vi "log analysis_gps.vi"() -> ()   [LabVIEW 2018] (continued)
-15.574401855,0.0,0.757817268,1.584750891,\"631T\",22,13,13,10,04,00,30,33*2671cfe0\n\tsystem status\tnormal 2 28.200000 0 0\trobot status\t31.566635\t41.045143\t9.231100\t-0.643525\t-0.931068\t52.416351\t0.448000\t-0.069000\n\t\n15:07:21.2\tlog_raw\tgps_raw\t#INSPVAXA,USB3,0,44.5,FINESTEERING,2107,281259.200,02000000,471d,15824;INS_ALIGNMENT_COMPLETE,INS_RTKFIXED,37.37050172881,126.72119309205,9.2293,22.3000,0.3645,0.2781,0.0053,-0.664590657,-1.103713757,34.708593103,0.4125,0.2928,0.5558,0.1115,0.0923,0.0801,0.2762,0.2590,5.0316,0f000001,0*10acd44c\n\tsystem status\tnormal 2 28.200000 0 0\trobot status\t31.709898\t41.234302\t9.229300\t-0.664591\t-1.103714\t53.022839\t0.470000\t-0.036000\n\t\n15:07:21.7\tlog_raw\tgps_raw\t#DUALANTENNAHEADINGA,USB3,0,44.5,FINESTEERING,2107,281259.700,02000000,d426,15824;SOL_COMPUTED,NARROW_INT,-1.000000000,37.724102020,-13.091491699,0.0,0.801039636,1.911924362,\"631T\",23,13,13,10,04,00,30,33*9a10e697\n\tsystem status\tnormal 2 28.200000 0 0\trobot status\t31.851856\t41.417794\t9.226400\t-0.835743\t-0.958959\t52.275898\t0.582000\t0.104000\n\t\n15:07:22.2\tlog_raw\tgps_raw\t#DUALANTENNAHEADINGA,USB3,0,46.0,FINESTEERING,2107,281260.200,02000000,d426,15824;SOL_COMPUTED,NARROW_INT,-1.000000000,39.115306854,-14.136718750,0.0,0.803064227,1.840907216,\"631T\",22,13,13,10,04,00,30,33*b50651c8\n\tsystem status\tnormal 2 28.200000 0 0\trobot status\t31.998440\t41.599620\t9.220500\t-0.986235\t-0.919071\t50.884693\t0.455000\t-0.083000\n\t\n15:07:22.7\tlog_raw\tgps_raw\t#INSPVAXA,USB3,0,46.0,FINESTEERING,2107,281260.700,02000000,471d,15824;INS_ALIGNMENT_COMPLETE,INS_RTKFIXED,37.37050659731,126.72119803894,9.2129,22.3000,0.3476,0.2954,-0.0046,-0.736337241,-0.866215786,36.967370061,0.4129,0.2931,0.5580,0.1111,0.0922,0.0796,0.2761,0.2587,5.0324,0f000001,0*f680867e\n\tsystem status\tnormal 2 28.200000 0 0\trobot status\t32.148086\t41.774629\t9.212900\t-0.736337\t-0.866216\t50.520088\t0.373000\t-0.188000\n\t\n15:07:23.2\tlog_raw\tgps_raw\t#DUALANTENNAHEADINGA,USB3,0,47.0,FINESTEERING,2107,281261.200,02000000,d426,15824;SOL_COMPUTED,NARROW_INT,-1.000000000,40.638893127,-14.791442871,0.0,0.948415875,1.839464903,\"631T\",22,13,13,10,04,00,30,33*e03d9ee2\n\tsystem status\tnormal 2 28.200000 0 0\trobot status\t32.299493\t41.952653\t9.205900\t-0.997560\t-1.091665\t49.361107\t0.437000\t-0.086000\n\t\n15:07:23.7\tlog_raw\tgps_raw\t#DUALANTENNAHEADINGA,USB3,0,47.0,FINESTEERING,2107,281261.700,02000000,d426,15824;SOL_COMPUTED,NARROW_INT,-1.000000000,41.109539032,-15.221740723,0.0,0.905525208,1.730005383,\"631T\",23,13,13,10,04,00,30,33*024d4917\n\tsystem status\tnormal 2 28.200000 0 0\trobot status\t32.455230\t42.129270\t9.201000\t-0.840900\t-1.049575\t48.890461\t0.564000\t0.092000\n\t\n15:07:24.2\tlog_raw\tgps_raw\t#INSPVAXA,USB3,0,48.5,FINESTEERING,2107,281262.200,02000000,471d,15824;INS_ALIGNMENT_COMPLETE,INS_RTKFIXED,37.37051135322,126.72120322169,9.1946,22.3000,0.3493,0.3226,-0.0187,-1.003564380,-0.949445467,38.532803613,0.4120,0.2907,0.5583,0.1108,0.0918,0.0785,0.2758,0.2584,5.0341,0f000001,0*bc77f761\n\tsystem status\tnormal 2 28.200000 0 0\trobot status\t32.607165\t42.302460\t9.194600\t-1.003564\t-0.949445\t48.849819\t0.509000\t0.011000\n\t\n15:07:24.7\tlog_raw\tgps_raw\t#DUALANTENNAHEADINGA,USB3,0,48.5,FINESTEERING,2107,281262.700,02000000,d426,15824;SOL_COMPUTED,NARROW_INT,-1.000000000,41.024471283,-13.771057129,0.0,0.941205680,1.970374942,\"631T\",22,13,13,10,04,00,30,33*2b107b4d\n\tsystem status\tnormal 2 28.200000 0 0\trobot status\t32.758480\t42.472024\t9.185100\t-0.965498\t-1.104615\t48.975529\t0.471000\t-0.009000\n\t\n15:07:25.2\tlog_raw\tgps_raw\t#INSPVAXA,USB3,0,45.5,FINESTEERING,2107,281263.200,02000000,471d,15824;INS_ALIGNMENT_COMPLETE,INS_RTKFIXED,37.37051438675,126.72120667905,9.1791,22.3000,0.3385,0.3277,0.0132,-0.749117776,-1.036053021,39.114622535,0.4097,0.2867,0.5508,0.1108,0.0917,0.0777,0.2757,0.2582,5.0350,0f000001,0*900f5f81\n\tsystem status\tnormal 2 28.200000 0 0\trobot status\t32.913413\t42.639134\t9.179100\t-0.749118\t-1.036053\t48.444920\t0.503000\t0.007000\n\t\n15:07:25.7\tlog_raw\tgps_raw\t#INSPVAXA,USB3,0,45.5,FINESTEERING,2107,281263.700,02000000,471d,15824;INS_ALIGNMENT_COMPLETE,INS_RTKFIXED,37.37051592724,126.72120843066,9.1725,22.3000,0.3345,0.3100,-0.0269,-0.953062315,-1.001119813,39.367076268,0.4097,0.2867,0.5508,0.1108,0.0917,0.0777,0.2757,0.2582,5.0350,0f000001,0*3f1ff118\n\tsystem status\tnormal 2 28.200000 0 0\trobot status\t33.068567\t42.810104\t9.172500\t-0.953062\t-1.001120\t48.758610\t0.495000\t0.014000\n\t\n15:07:26.2\tlog_raw\tgps_raw\t#DUALANTENNAHEADINGA,USB3,0,45.5,FINESTEERING,2107,281264.200,02000000,d426,15824;SOL_COMPUTED,NARROW_INT,-1.000000000,41.910186768,-13.638671875,0.0,0.987370729,2.013862848,\"631T\",24,13,13,10,04,00,30,33*886cbc18\n\tsystem status\tnormal 2 28.200000 0 0\trobot status\t33.222421\t42.973971\t9.165800\t-0.908836\t-0.953888\t48.089813\t0.490000\t0.012000\n\t\n15:07:26.7\tlog_raw\tgps_raw\t#DUALANTENNAHEADINGA,USB3,0,45.5,FINESTEERING,2107,281264.700,02000000,d426,15824;SOL_COMPUTED,NARROW_INT,-1.000000000,42.165882111,-13.191467285,0.0,1.231637120,2.283805132,\"631T\",23,11,11,8,04,00,30,03*d347cf5b\n\tsystem status\tnormal 2 28.200000 0 0\trobot status\t33.385986\t43.147920\t9.157400\t-0.806230\t-0.977712\t47.834118\t0.498000\t0.015000\n\t\n15:07:27.2\tlog_raw\tgps_raw\t#DUALANTENNAHEADINGA,USB3,0,48.5,FINESTEERING,2107,281265.200,02000000,d426,15824;SOL_COMPUTED,NARROW_INT,-1.000000000,41.782566071,-14.026184082,0.0,0.949394464,1.456767678,\"631T\",24,12,12,8,04,00,30,03*b5e68f03\n\tsystem status\tnormal 2 28.300000 0 0\trobot status\t33.551266\t43.323593\t9.149800\t-0.943344\t-1.087324\t48.217434\t0.504000\t0.015000\n\t\n15:07:27.7\tlog_raw\tgps_raw\t#DUALANTENNAHEADINGA,USB3,0,48.5,FINESTEERING,2107,281265.700,02000000,d426,15824;SOL_COMPUTED,NARROW_INT,-1.000000000,42.654987335,-13.940582275,0.0,0.905997872,1.456194401,\"631T\",25,12,12,8,04,00,30,03*ebbb69a1\n\tsystem status\tnormal 2 28.200000 0 0\trobot status\t33.713510\t43.493528\t9.144600\t-0.914763\t-1.022784\t47.345013\t0.602000\t-0.140000\n\t\n15:07:28.2\tlog_raw\tgps_raw\t#DUALANTENNAHEADINGA,USB3,0,44.0,FINESTEERING,2107,281266.200,02000000,d426,15824;SOL_COMPUTED,NARROW_INT,-1.000000000,41.473289490,-13.976562500,0.0,0.876108646,1.437642574,\"631T\",26,12,12,8,04,00,30,03*9c4cfbf2\n\tsystem status\tnormal 2 28.100000 0 0\trobot status\t33.872849\t43.664287\t9.139200\t-0.953588\t-0.975012\t48.526711\t0.573000\t-0.084000\n\t\n15:07:28.7\tlog_raw\tgps_raw\t#INSPVAXA,USB3,0,44.0,FINESTEERING,2107,281266.700,02000000,471d,15824;INS_ALIGNMENT_COMPLETE,INS_RTKFIXED,37.37052514721,126.72121924696,9.1351,22.3000,0.3260,0.3161,-0.0126,-0.947375074,-0.706024295,38.522505124,0.4363,0.2885,0.5509,0.1172,0.0950,0.0803,0.2752,0.2577,5.0353,0f000001,0*ab36857c\n\tsystem status\tnormal 2 28.000000 0 0\trobot status\t34.026658\t43.833375\t9.135100\t-0.947375\t-0.706024\t48.338646\t0.361000\t0.243000\n\t\n15:07:29.2\tlog_raw\tgps_raw\t#DUALANTENNAHEADINGA,USB3,0,48.0,FINESTEERING,2107,281267.200,02000000,d426,15824;SOL_COMPUTED,NARROW_INT,-1.000000000,40.023796082,-13.769653320,0.0,1.105050921,2.107353687,\"631T\",22,12,12,8,04,00,30,03*89f55c6d\n\tsystem status\tnormal 2 28.000000 0 0\trobot status\t34.180182\t44.006389\t9.131600\t-0.895036\t-0.801690\t49.976204\t0.562000\t-0.071000\n\t\n15:07:29.7\tlog_raw\tgps_raw\t#DUALANTENNAHEADINGA,USB3,0,48.0,FINESTEERING,2107,281267.700,02000000,d426,15824;SOL_COMPUTED,NARROW_INT,-1.000000000,38.975990295,-14.866943359,0.0,1.019285679,1.869416475,\"631T\",22,12,12,8,04,00,30,03*a0488b34\n\tsystem status\tnormal 2 28.000000 0 0\trobot status\t34.334172\t44.181531\t9.127500\t-0.727606\t-0.705041\t51.024010\t0.354000\t0.251000\n\t\n15:07:30.2\tlog_raw\tgps_raw\t#DUALANTENNAHEADINGA,USB3,0,48.0,FINESTEERING,2107,281268.200,02000000,d426,15824;SOL_COMPUTED,NARROW_INT,-1.000000000,37.457145691,-14.142669678,0.0,0.916966915,1.645377994,\"631T\",25,12,12,8,04,00,30,03*51ae3b94\n\tsystem status\tnormal 2 28.000000 0 0\trobot status\t34.484633\t44.363511\t9.124000\t-0.782242\t-1.013218\t52.542854\t0.617000\t-0.117000\n\t\n15:07:30.7\tlog_raw\tgps_raw\t#DUALANTENNAHEADINGA,USB3,0,48.0,FINESTEERING,2107,281268.700,02000000,d426,15824;SOL_COMPUTED,NARROW_INT,-1.000000000,36.570995331,-12.889495850,0.0,0.874405205,1.610776067,\"631T\",27,12,12,8,04,00,30,03*59172eb5\n\tsystem status\tnormal 2 28.000000 0 0\trobot status\t34.629130\t44.546597\t9.120400\t-0.707911\t-0.956168\t53.429005\t0.665000\t-0.257000\n\t\n15:07:31.2\tlog_raw\tgps_raw\t#DUALANTENNAHEADINGA,USB3,0,43.5,FINESTEERING,2107,281269.200,02000000,d426,15824;SOL_COMPUTED,NARROW_INT,-1.000000000,35.973979950,-14.332061768,0.0,0.830094159,1.497864485,\"631T\",27,12,12,8,04,00,30,03*090ddc0d\n\tsystem status\tnormal 2 28.100000 0 0\trobot status\t34.770052\t44.733261\t9.118400\t-0.795683\t-0.850425\t54.026020\t0.605000\t-0.143000\n\t\n15:07:31.7\tlog_raw\tgps_raw\t#DUALANTENNAHEADINGA,USB3,0,43.5,FINESTEERING,2107,281269.700,02000000,d426,15824;SOL_COMPUTED,NARROW_INT,-1.000000000,35.818984985,-16.138092041,0.0,0.812042832,1.471114397,\"631T\",26,12,12,8,04,00,30,03*f4bb3c31\n\tsystem status\tnormal 2 28.100000 0 0\trobot status\t34.908478\t44.923072\t9.116600\t-0.660770\t-0.782310\t54.181015\t0.442000\t0.104000\n\t\n15:07:32.2\tlog_raw\tgps_raw\t#DUALANTENNAHEADINGA,USB3,0,46.5,FINESTEERING,2107,281270.200,02000000,d426,15824;SOL_COMPUTED,NARROW_INT,-1.000000000,35.621791840,-13.436737061,0.0,0.778346181,1.418952346,\"631T\",25,12,12,8,04,00,30,03*c6e6dbb2\n\tsystem status\tnormal 2 28.100000 0 0\trobot status\t35.047785\t45.119572\t9.114200\t-0.835759\t-0.956556\t54.378208\t0.421000\t0.108000\n\t\n15:07:32.7\tlog_raw\tgps_raw\t#DUALANTENNAHEADINGA,USB3,0,46.5,FINESTEERING,2107,281270.700,02000000,d426,15824;SOL_COMPUTED,NARROW_INT,-1.000000000,35.070240021,-13.728149414,0.0,0.744003534,1.356679201,\"631T\",25,12,12,8,04,00,30,03*cf10d1c9\n\tsystem status\tnormal 2 28.200000 0 0\trobot status\t35.184021\t45.314772\t9.112900\t-0.827370\t-0.902708\t54.929760\t0.608000\t-0.143000\n\t\n15:07:33.2\tlog_raw\tgps_raw\t#DUALANTENNAHEADINGA,USB3,0,45.5,FINESTEERING,2107,281271.200,02000000,d426,15824;SOL_COMPUTED,NARROW_INT,-1.000000000,35.494377136,-13.422943115,0.0,0.983616889,2.186612129,\"631T\",23,12,12,8,04,00,30,03*afbd86f5\n\tsystem status\tnormal 2 28.200000 0 0\trobot status\t35.321899\t45.512581\t9.111000\t-0.616810\t-0.962309\t54.505623\t0.386000\t0.164000\n\t\n15:07:33.7\tlog_raw\tgps_raw\t#DUALANTENNAHEADINGA,USB3,0,45.5,FINESTEERING,2107,281271.700,02000000,d426,15824;SOL_COMPUTED,NARROW_INT,-1.000000000,35.115871429,-12.229492188,0.0,0.917624831,2.129554033,\"631T\",22,11,11,8,04,00,30,03*47d1ca67\n\tsystem status\tnormal 2 28.200000 0 0\trobot status\t35.456033\t45.711150\t9.110300\t-0.770202\t-0.898350\t54.884129\t0.467000\t0.040000\n\t\n15:07:34.2\tlog_raw\tgps_raw\t#DUALANTENNAHEADINGA,USB3,0,45.0,FINESTEERING,2107,281272.200,02000000,d426,15824;SOL_COMPUTED,NARROW_INT,-1.000000000,35.165107727,-13.680572510,0.0,0.853601813,1.895400286,\"631T\",23,11,11,8,04,00,30,03*664b8012\n\tsystem status\tnormal 2 28.200000 0 0\trobot status\t35.595153\t45.913396\t9.108200\t-0.692435\t-1.007162\t54.834892\t0.467000\t0.023000\n\t\n15:07:34.7\tlog_raw\tgps_raw\t#DUALANTENNAHEADINGA,USB3,0,45.0,FINESTEERING,2107,281272.700,02000000,d426,15824;SOL_COMPUTED,NARROW_INT,-1.000000000,35.308296204,-13.433410645,0.0,0.833106577,1.789978504,\"631T\",23,11,11,8,04,00,30,03*efeaf6da\n\tsystem status\tnormal 2 28.200000 0 0\trobot status\t35.734434\t46.115790\t9.102900\t-0.678981\t-1.146702\t54.691704\t0.482000\t0.009000\n\t\n15:07:35.2\tlog_raw\tgps_raw\t#DUALANTENNAHEADINGA,USB3,0,46.0,FINESTEERING,2107,281273.200,02000000,d426,15824;SOL_COMPUTED,NARROW_INT,-1.000000000,36.192741394,-16.037811279,0.0,0.810550869,1.694264531,\"631T\",22,11,11,8,04,00,30,03*4456d48d\n\tsystem status\tnormal 2 28.200000 0 0\trobot status\t35.871255\t46.311320\t9.099300\t-0.536086\t-1.483888\t53.807259\t0.505000\t-0.028000\n\t\n15:07:35.7\tlog_raw\tgps_raw\t\tsystem status\tnormal 2 28.200000 0 0\trobot status\t36.007822\t46.507939\t9.097500\t-0.602065\t-1.516155\t53.983997\t0.489000\t-0.023000\n\t\n15:07:36.2\tlog_raw\tgps_raw\t#DUALANTENNAHEADINGA,USB3,0,48.0,FINESTEERING,2107,281274.200,02000000,d426,15824;SOL_COMPUTED,NARROW_INT,-1.000000000,35.622310638,-14.246795654,0.0,1.186534643,2.124257803,\"631T\",23,13,13,10,04,00,30,33*4699dedc\n\tsystem status\tnormal 2 28.200000 0 0\trobot status\t36.147250\t46.710270\t9.090800\t-0.727838\t-1.235927\t54.377689\t0.492000\t-0.015000\n\t\n15:07:36.7\tlog_raw\tgps_raw\t\tsystem status\tnormal 2 28.300000 0 0\trobot status\t36.284167\t46.907030\t9.084300\t-0.725999\t-1.253532\t54.463184\t0.493000\t-0.018000\n\t\n15:07:37.2\tlog_raw\tgps_raw\t#DUALANTENNAHEADINGA,USB3,0,45.0,FINESTEERING,2107,281275.200,02000000,d426,15824;SOL_COMPUTED,NARROW_INT,-1.000000000,35.922065735,-12.943084717,0.0,1.068319321,2.159161329,\"631T\",24,13,13,10,04,00,30,23*90535b08\n\tsystem status\tnormal 2 28.300000 0 0\trobot status\t36.415424\t47.091111\t9.080700\t-0.590725\t-1.108653\t54.077934\t0.494000\t-0.024000\n\t\n15:07:37.7\tlog_raw\tgps_raw\t#DUALANTENNAHEADINGA,USB3,0,45.0,FINESTEERING,2107,281275.700,02000000,d426,15824;SOL_COMPUTED,NARROW_INT,-1.000000000,35.806697845,-14.127471924,0.0,1.191707134,2.929863453,\"631T\",23,13,13,10,04,00,30,33*14f638f6\n\tsystem status\tnormal 2 28.200000 0 0\trobot status\t36.555534\t47.288330\t9.077900\t-0.847597\t-1.031601\t54.193302\t0.498000\t-0.035000\n\t\n15:07:38.2\tlog_raw\tgps_raw\t\tsystem status\tnormal 2 28.200000 0 0\trobot status\t36.697376\t47.486132\t9.075700\t-0.966277\t-0.867460\t53.488716\t0.476000\t-0.014000\n\t\n15:07:38.7\tlog_raw\tgps_raw\t\tsystem status\tnormal 2 28.200000 0 0\trobot status\t36.838734\t47.678234\t9.075000\t-0.743731\t-0.878510\t52.994225\t0.507000\t-0.012000\n\t\n15:07:39.2\tlog_raw\tgps_raw\t#DUALANTENNAHEADINGA,USB3,0,47.5,FINESTEERING,2107,281277.200,02000000,d426,15824;SOL_COMPUTED,NARROW_INT,-1.000000000,36.727424622,-13.082946777,0.0,0.949807763,2.157425642,\"631T\",23,11,11,8,04,00,30,03*dbda4352\n\tsystem status\tnormal 2 28.200000 0 0\trobot status\t36.981502\t47.872071\t9.074100\t-0.771341\t-0.814677\t53.272575\t0.497000\t-0.019000\n\t\n15:07:39.7\tlog_raw\tgps_raw\t\tsystem status\tnormal 2 28.200000 0 0\trobot status\t37.126902\t48.063305\t9.075700\t-0.664587\t-1.042074\t53.167221\t0.578000\t0.099000\n\t\n15:07:40.2\tlog_raw\tgps_raw\t#DUALANTENNAHEADINGA,USB3,0,47.0,FINESTEERING,2107,281278.200,02000000,d426,15824;SOL_COMPUTED,NARROW_INT,-1.000000000,38.801025391,-13.665405273,0.0,1.011600971,2.213801622,\"631T\",23,11,11,8,04,00,30,03*a2b4300d\n\tsystem status\tnormal 2 28.200000 0 0\trobot status\t37.270479\t48.250911\t9.075300\t-0.703013\t-0.987348\t51.198975\t0.484000\t-0.048000\n\t\n15:07:40.7\tlog_raw\tgps_raw\t\tsystem status\tnormal 2 28.200000 0 0\trobot status\t37.419608\t48.442360\t9.072100\t-0.758993\t-1.063474\t50.790871\t0.434000\t-0.124000\n\t\n15:07:41.2\tlog_raw\tgps_raw\t#DUALANTENNAHEADINGA,USB3,0,44.5,FINESTEERING,2107,281279.200,02000000,d426,15824;SOL_COMPUTED,NARROW_INT,-1.000000000,39.271907806,-13.744201660,0.0,0.885574758,1.866288543,\"631T\",24,11,11,8,04,00,30,03*14651a74\n\tsystem status\tnormal 2 28.200000 0 0\trobot status\t37.564073\t48.625273\t9.068400\t-0.756006\t-0.992828\t50.728092\t0.460000\t-0.070000\n\t\n15:07:41.7\tlog_raw\tgps_raw\t\tsystem status\tnormal 2 28.200000 0 0\trobot status\t37.713760\t48.813692\t9.062800\t-0.823894\t-1.057064\t50.037521\t0.395000\t-0.114000\n\t\n15:07:42.2\tlog_raw\tgps_raw\t\tsystem status\tnormal 2 28.200000 0 0\trobot status\t37.862921\t48.995193\t9.058900\t-0.752662\t-0.902912\t50.282597\t0.502000\t0.016000\n\t\n15:07:42.7\tlog_raw\tgps_raw\t#DUALANTENNAHEADINGA,USB3,0,48.0,FINESTEERING,2107,281280.700,02000000,d426,15824;SOL_COMPUTED,NARROW_INT,-1.000000000,40.700374603,-12.203552246,0.0,0.796584129,1.643284798,\"631T\",24,11,11,8,04,00,30,03*0355bfc3\n\tsystem status\tnormal 2 28.200000 0 0\trobot status\t38.015447\t49.176889\t9.058400\t-0.805111\t-0.901408\t49.299625\t0.476000\t-0.022000\n\t\n15:07:43.2\tlog_raw\tgps_raw\t\tsystem status\tnormal 2 28.200000 0 0\trobot status\t38.168522\t49.355987\t9.054400\t-0.980266\t-0.609275\t49.185120\t0.511000\t0.011000\n\t\n15:07:43.7\tlog_raw\tgps_raw\t#DUALANTENNAHEADINGA,USB3,0,43.5,FINESTEERING,2107,281281.700,02000000,d426,15824;SOL_COMPUTED,NARROW_INT,-1.000000000,41.025180817,-13.610565186,0.0,1.006764770,1.762146711,\"631T\",23,11,11,8,04,00,30,03*95eb9222\n\tsystem status\tnormal 2 28.200000 0 0\trobot status\t38.323525\t49.525802\t9.048900\t-0.595366\t-0.860197\t48.974819\t0.485000\t0.004000\n\t\n15:07:44.2\tlog_raw\tgps_raw\t\tsystem status\tnormal 2 28.200000 0 0\trobot status\t38.479198\t49.700891\t9.045700\t-0.786808\t-0.739360\t47.852482\t0.490000\t0.014000\n\t\n15:07:44.7\tlog_raw\tgps_raw\t#DUALANTENNAHEADINGA,USB3,0,48.5,FINESTEERING,2107,281282.700,02000000,d426,15824;SOL_COMPUTED,NARROW_INT,-1.000000000,42.471115112,-14.988128662,0.0,1.268621087,2.738634586,\"631T\",23,13,13,9,04,00,20,23*7676e672\n\tsystem status\tnormal 2 28.200000 0 0\trobot status\t38.628012\t49.869703\t9.041100\t-1.082338\t-0.662611\t47.528885\t0.491000\t0.015000\n\t\n15:07:45.2\tlog_raw\tgps_raw\t#INSPVAXA,USB3,0,48.0,FINESTEERING,2107,281283.250,02000000,471d,15824;INS_ALIGNMENT_COMPLETE,INS_RTKFIXED,37.37058125614,126.72127316558,9.0365,22.3000,0.3478,0.3335,-0.0027,-0.704403404,-0.836236554,39.118701803,0.4319,0.3133,0.6216,0.1204,0.1024,0.0974,0.2734,0.2534,5.0561,0f000001,0*0df7e601\n\tsystem status\tnormal 2 28.200000 0 0\trobot status\t38.802681\t50.060581\t9.036500\t-0.704403\t-0.836237\t48.533897\t0.502000\t0.030000\n\t\n15:07:45.7\tlog_raw\tgps_raw\t#DUALANTENNAHEADINGA,USB3,0,48.0,FINESTEERING,2107,281283.700,02000000,d426,15824;SOL_COMPUTED,NARROW_INT,-1.000000000,41.292312622,-13.761383057,0.0,1.487377644,3.398363352,\"631T\",25,10,10,8,04,00,30,03*49b52b61\n\tsystem status\tnormal 2 28.200000 0 0\trobot status\t38.946357\t50.221947\t9.035600\t-0.938084\t-0.748688\t48.707687\t0.500000\t0.017000\n\t\n15:07:46.2\tlog_raw\tgps_raw\t#INSPVAXA,USB3,0,44.5,FINESTEERING,2107,281284.250,02000000,471d,15824;INS_ALIGNMENT_COMPLETE,INS_RTKFIXED,37.37058446322,126.72127677415,9.0328,22.3000,0.3259,0.3273,-0.0037,-0.937814691,-0.658439283,39.092377906,0.4304,0.3133,0.6248,0.1182,0.0996,0.0951,0.2734,0.2534,5.0568,0f000001,0*6df0d0a0\n\tsystem status\tnormal 2 28.200000 0 0\trobot status\t39.122322\t50.416516\t9.032800\t-0.937815\t-0.658439\t49.048512\t0.434000\t0.108000\n\t\n15:07:46.7\tlog_raw\tgps_raw\t\tsystem status\tnormal 2 28.100000 0 0\trobot status\t39.265720\t50.576645\t9.028100\t-0.931821\t-0.651062\t48.507782\t0.516000\t-0.019000\n\t\n15:07:47.2\tlog_raw\tgps_raw\t#DUALANTENNAHEADINGA,USB3,0,45.0,FINESTEERING,2107,281285.200,02000000,d426,15824;SOL_COMPUTED,NARROW_INT,-1.000000000,40.100524902,-11.947021484,0.0,1.414593220,3.733982325,\"631T\",25,10,10,8,04,00,30,03*9b9ac519\n\tsystem status\tnormal 2 28.100000 0 0\trobot status\t39.418438\t50.753731\t9.026400\t-1.045904\t-0.622362\t49.899475\t0.367000\t0.232000\n\t\n15:07:47.7\tlog_raw\tgps_raw\t#INSPVAXA,USB3,0,45.0,FINESTEERING,2107,281285.750,02000000,471d,15824;INS_ALIGNMENT_COMPLETE,INS_RTKFIXED,37.37058925318,126.72128198037,9.0239,22.3000,0.3334,0.2935,0.0143,-0.808488626,-0.666784324,37.099598741,0.4334,0.3188,0.6428,0.1170,0.0987,0.0941,0.2735,0.2534,5.0574,0f000001,0*332dca9d\n\tsystem status\tnormal 2 28.100000 0 0\trobot status\t39.583480\t50.948126\t9.023900\t-0.808489\t-0.666784\t50.980686\t0.340000\t0.231000\n\t\n15:07:48.2\tlog_raw\tgps_raw\t\tsystem status\tnormal 2 28.000000 0 0\trobot status\t39.716456\t51.111886\t9.021500\t-0.669660\t-0.741115\t51.504147\t0.461000\t0.100000\n\t\n15:07:48.7\tlog_raw\tgps_raw\t#DUALANTENNAHEADINGA,USB3,0,47.0,FINESTEERING,2107,281286.700,02000000,d426,15824;SOL_COMPUTED,NARROW_INT,-1.000000000,38.718589783,-13.239685059,0.0,1.092944860,2.696835995,\"631T\",24,10,10,8,04,00,30,03*03484901\n\tsystem status\tnormal 2 28.000000 0 0\trobot status\t39.859819\t51.303062\t9.018200\t-0.911625\t-1.044323\t51.281410\t0.609000\t-0.142000\n\t\n15:07:49.2\tlog_raw\tgps_raw\t\tsystem status\tnormal 2 28.000000 0 0\trobot status\t39.998635\t51.492159\t9.013800\t-0.809440\t-1.050845\t52.888622\t0.391000\t0.170000\n\t\n15:07:49.7\tlog_raw\tgps_raw\t#DUALANTENNAHEADINGA,USB3,0,47.0,FINESTEERING,2107,281287.700,02000000,d426,15824;SOL_COMPUTED,NARROW_INT,-1.000000000,36.104297638,-13.498443604,0.0,0.922848761,2.195329189,\"631T\",26,10,10,8,04,00,30,03*04480a52\n\tsystem status\tnormal 2 28.100000 0 0\trobot status\t40.135370\t51.683837\t9.009000\t-0.800921\t-0.896046\t53.895702\t0.367000\t0.224000\n\t\n15:07:50.2\tlog_raw\tgps_raw\t#INSPVAXA,USB3,0,47.5,FINESTEERING,2107,281288.250,02000000,471d,15824;INS_ALIGNMENT_COMPLETE,INS_RTKFIXED,37.37059781001,126.72128984433,9.0038,22.3000,0.3744,0.2594,-0.0022,-0.807848341,-0.697649833,32.607000206,0.4351,0.3197,0.6721,0.1156,0.0982,0.0924,0.2733,0.2531,5.0607,0f000001,0*7ad3d381\n\tsystem status\tnormal 2 28.100000 0 0\trobot status\t40.280057\t51.897799\t9.003800\t-0.807848\t-0.697650\t53.988251\t0.428000\t0.116000\n\t\n15:07:50.7\tlog_raw\tgps_raw\t#DUALANTENNAHEADINGA,USB3,0,47.5,FINESTEERING,2107,281288.700,02000000,d426,15824;SOL_COMPUTED,NARROW_INT,-1.000000000,34.380798340,-12.289306641,0.0,0.881599903,2.027381897,\"631T\",24,10,10,8,04,00,30,03*fd23ace1\n\tsystem status\tnormal 2 28.100000 0 0\trobot status\t40.398568\t52.080059\t8.999400\t-0.727871\t-0.931697\t55.619202\t0.598000\t-0.139000\n\t\n15:07:51.2\tlog_raw\tgps_raw\t#INSPVAXA,USB3,0,43.0,FINESTEERING,2107,281289.250,02000000,471d,15824;INS_ALIGNMENT_COMPLETE,INS_RTKFIXED,37.37060144846,126.72129278207,8.9959,22.3000,0.3637,0.2540,-0.0055,-0.784801364,-1.198337190,31.676492197,0.4344,0.3185,0.6737,0.1148,0.0977,0.0905,0.2732,0.2529,5.0623,0f000001,0*0e64d244\n\tsystem status\tnormal 2 28.100000 0 0\trobot status\t40.540277\t52.301609\t8.995900\t-0.784801\t-1.198337\t55.390762\t0.568000\t-0.112000\n\t\n15:07:51.7\tlog_raw\tgps_raw\t\tsystem status\tnormal 2 28.200000 0 0\trobot status\t40.656983\t52.485859\t8.990900\t-0.841622\t-1.206879\t55.521332\t0.426000\t0.109000\n\t\n15:07:52.2\tlog_raw\tgps_raw\t#DUALANTENNAHEADINGA,USB3,0,47.0,FINESTEERING,2107,281290.200,02000000,d426,15824;SOL_COMPUTED,NARROW_INT,-1.000000000,34.493209839,-14.783813477,0.0,0.972535849,1.987741113,\"631T\",22,10,10,8,04,00,30,03*2d07aef6\n\tsystem status\tnormal 2 28.200000 0 0\trobot status\t40.786858\t52.689235\t8.985800\t-0.708265\t-1.382941\t55.506790\t0.550000\t-0.106000\n\t\n15:07:52.7\tlog_raw\tgps_raw\t\tsystem status\tnormal 2 28.200000 0 0\trobot status\t40.919320\t52.896058\t8.981700\t-0.619521\t-1.535397\t55.462795\t0.462000\t0.033000\n\t\n15:07:53.2\tlog_raw\tgps_raw\t#INSPVAXA,USB3,0,47.0,FINESTEERING,2107,281291.250,02000000,471d,15824;INS_ALIGNMENT_COMPLETE,INS_RTKFIXED,37.37060884718,126.72129871265,8.9767,22.3000,0.3938,0.2598,0.0143,-0.672164734,-1.279451684,31.580297519,0.4248,0.3046,0.6381,0.1143,0.0969,0.0864,0.2729,0.2527,5.0655,0f000001,0*eac27b45\n\tsystem status\tnormal 2 28.200000 0 0\trobot status\t41.065598\t53.122751\t8.976700\t-0.672165\t-1.279452\t55.013996\t0.503000\t-0.018000\n\t\n15:07:53.7\tlog_raw\tgps_raw\t\tsystem status\tnormal 2 28.200000 0 0\trobot status\t41.180313\t53.298203\t8.973400\t-0.877294\t-1.135816\t54.990143\t0.474000\t0.003000\n\t\n15:07:54.2\tlog_raw\tgps_raw\t#INSPVAXA,USB3,0,48.0,FINESTEERING,2107,281292.250,02000000,471d,15824;INS_ALIGNMENT_COMPLETE,INS_RTKFIXED,37.37061243778,126.72130169584,8.9693,22.3000,0.3929,0.2526,0.0002,-0.566566315,-1.022014825,31.866570439,0.4222,0.3014,0.6236,0.1151,0.0976,0.0859,0.2728,0.2526,5.0668,0f000001,0*f1faa83c\n\tsystem status\tnormal 2 28.200000 0 0\trobot status\t41.329844\t53.521251\t8.969300\t-0.566566\t-1.022015\t54.607853\t0.494000\t-0.018000\n\t\n15:07:54.7\tlog_raw\tgps_raw\t\tsystem status\tnormal 2 28.200000 0 0\trobot status\t41.448026\t53.700928\t8.965600\t-0.554965\t-1.221563\t55.514385\t0.495000\t-0.016000\n\t\n15:07:55.2\tlog_raw\tgps_raw\t#INSPVAXA,USB3,0,46.5,FINESTEERING,2107,281293.250,02008000,471d,15824;INS_ALIGNMENT_COMPLETE,INS_RTKFIXED,37.37061609007,126.72130472150,8.9616,22.3000,0.3940,0.2710,0.0085,-0.635134028,-1.458627956,32.227180658,0.4201,0.2993,0.6101,0.1147,0.0971,0.0842,0.2727,0.2523,5.0683,0f000001,0*f561f230\n\tsystem status\tnormal 2 28.200000 0 0\trobot status\t41.597852\t53.926597\t8.961600\t-0.635134\t-1.458628\t55.285629\t0.495000\t-0.018000\n\t\n15:07:55.7\tlog_raw\tgps_raw\t\tsystem status\tnormal 2 28.200000 0 0\trobot status\t41.717377\t54.101745\t8.958300\t-0.727505\t-1.117508\t55.508831\t0.490000\t-0.016000\n\t\n15:07:56.2\tlog_raw\tgps_raw\t#INSPVAXA,USB3,0,44.0,FINESTEERING,2107,281294.250,02008000,471d,15824;INS_ALIGNMENT_COMPLETE,INS_RTKFIXED,37.37061971209,126.72130780942,8.9541,22.3000,0.4211,0.2805,-0.0013,-0.831057528,-0.973116306,32.803325503,0.4188,0.2977,0.5988,0.1153,0.0975,0.0844,0.2725,0.2520,5.0696,0f000001,0*1928a823\n\tsystem status\tnormal 2 28.200000 0 0\trobot status\t41.871375\t54.328584\t8.954100\t-0.831058\t-0.973116\t54.554722\t0.492000\t-0.026000\n\t\n15:07:56.7\tlog_raw\tgps_raw\t#INSPVAXA,USB3,0,44.0,FINESTEERING,2107,281294.750,02008000,471d,15824;INS_ALIGNMENT_COMPLETE,INS_RTKFIXED,37.37062151019,126.72130936764,8.9520,22.3000,0.3975,0.2634,0.0090,-0.724790685,-1.060395947,33.026627760,0.4188,0.2977,0.5988,0.1153,0.0975,0.0844,0.2725,0.2520,5.0696,0f000001,0*daa7d020\n\tsystem status\tnormal 2 28.200000 0 0\trobot status\t42.009400\t54.528145\t8.952000\t-0.724791\t-1.060396\t54.415871\t0.495000\t-0.025000\n\t\n15:07:57.2\tlog_raw\tgps_raw\t#INSPVAXA,USB3,0,48.0,FINESTEERING,2107,281295.250,02008000,471d,15824;INS_ALIGNMENT_COMPLETE,INS_RTKFIXED,37.37062331676,126.72131094056,8.9508,22.3000,0.4136,0.2984,0.0031,-0.941558155,-1.233075222,33.345568477,0.4178,0.2964,0.5888,0.1164,0.0983,0.0857,0.2723,0.2516,5.0710,0f000001,0*4b91ac30\n\tsystem status\tnormal 2 28.200000 0 0\trobot status\t42.148726\t54.728646\t8.950800\t-0.941558\t-1.233075\t54.361309\t0.492000\t-0.016000\n\t\n15:07:57.7\tlog_raw\tgps_raw\t#INSPVAXA,USB3,0,48.0,FINESTEERING,2107,281295.750,02008000,471d,15824;INS_ALIGNMENT_COMPLETE,INS_RTKFIXED,37.37062507494,126.72131254716,8.9509,22.3000,0.4055,0.2849,-0.0018,-0.776132833,-1.125745955,33.718162525,0.4178,0.2964,0.5888,0.1164,0.0983,0.0857,0.2723,0.2516,5.0710,0f000001,0*fb568b3d\n\tsystem status\tnormal 2 28.200000 0 0\trobot status\t42.291036\t54.923776\t8.950900\t-0.776133\t-1.125746\t53.586090\t0.505000\t-0.016000\n\t\n15:07:58.2\tlog_raw\tgps_raw\t\tsystem status\tnormal 2 28.200000 0 0\trobot status\t42.419876\t55.099393\t8.950200\t-0.725828\t-1.060978\t53.230602\t0.498000\t-0.023000\n\t\n15:07:58.7\tlog_raw\tgps_raw\t#INSPVAXA,USB3,0,46.0,FINESTEERING,2107,281296.750,02008000,471d,15824;INS_ALIGNMENT_COMPLETE,INS_RTKFIXED,37.37062859977,126.72131581022,8.9479,22.3000,0.4084,0.2870,-0.0048,-0.626858004,-1.220047276,34.496993035,0.4174,0.2953,0.5808,0.1166,0.0980,0.0866,0.2720,0.2512,5.0719,0f000001,0*b70d9a1a\n\tsystem status\tnormal 2 28.200000 0 0\trobot status\t42.580073\t55.314976\t8.947900\t-0.626858\t-1.220047\t52.350243\t0.492000\t-0.024000\n\t\n15:07:59.2\tlog_raw\tgps_raw\t\tsystem status\tnormal 2 28.200000 0 0\trobot status\t42.709665\t55.485973\t8.946000\t-0.724943\t-0.913191\t51.877937\t0.504000\t-0.019000\n\t\n15:07:59.7\tlog_raw\tgps_raw\t#INSPVAXA,USB3,0,46.5,FINESTEERING,2107,281297.750,02000000,471d,15824;INS_ALIGNMENT_COMPLETE,INS_RTKFIXED,37.37063201269,126.72131910032,8.9415,22.3000,0.3858,0.2920,-0.0049,-0.857107455,-1.040274472,35.314316198,0.4170,0.2951,0.5749,0.1163,0.0975,0.0871,0.2718,0.2508,5.0734,0f000001,0*148bd1ed\n\tsystem status\tnormal 2 28.300000 0 0\trobot status\t42.871505\t55.693757\t8.941500\t-0.857107\t-1.040274\t51.127346\t0.541000\t0.060000\n\t\n15:08:00.2\tlog_raw\tgps_raw\t#INSPVAXA,USB3,0,47.5,FINESTEERING,2107,281298.250,02000000,471d,15824;INS_ALIGNMENT_COMPLETE,INS_RTKFIXED,37.37063371305,126.72132080320,8.9374,22.3000,0.3749,0.3041,0.0076,-0.820490736,-1.287497218,35.568330559,0.4168,0.2950,0.5704,0.1159,0.0968,0.0877,0.2716,0.2505,5.0751,0f000001,0*0458b711\n\tsystem status\tnormal 2 28.200000 0 0\trobot status\t43.022343\t55.882470\t8.937400\t-0.820491\t-1.287497\t52.237698\t0.484000\t-0.013000\n\t\n15:08:00.7\tlog_raw\tgps_raw\t\tsystem status\tnormal 2 28.200000 0 0\trobot status\t43.152336\t56.043862\t8.935300\t-0.982494\t-1.398492\t50.827724\t0.480000\t-0.007000\n\t\n15:08:01.2\tlog_raw\tgps_raw\t#INSPVAXA,USB3,0,48.0,FINESTEERING,2107,281299.250,02000000,471d,15824;INS_ALIGNMENT_COMPLETE,INS_RTKFIXED,37.37063695179,126.72132414290,8.9320,22.3000,0.3767,0.2972,0.0004,-0.739787726,-1.092581403,36.370475984,0.4162,0.2936,0.5661,0.1155,0.0962,0.0881,0.2714,0.2503,5.0767,0f000001,0*980b2911\n\tsystem status\tnormal 2 28.200000 0 0\trobot status\t43.318168\t56.241918\t8.932000\t-0.739788\t-1.092581\t51.898197\t0.494000\t-0.011000\n\t\n15:08:01.7\tlog_raw\tgps_raw\t#INSPVAXA,USB3,0,48.0,FINESTEERING,2107,281299.750,02000000,471d,15824;INS_ALIGNMENT_COMPLETE,INS_RTKFIXED,37.37063857725,126.72132585702,8.9270,22.3000,0.3719,0.3148,0.0043,-0.737895433,-1.223503382,36.673164573,0.4162,0.2936,0.5661,0.1155,0.0962,0.0881,0.2714,0.2503,5.0767,0f000001,0*b3e17f59\n\tsystem status\tnormal 2 28.200000 0 0\trobot status\t43.470002\t56.422319\t8.927000\t-0.737895\t-1.223503\t51.044170\t0.499000\t0.000000\n\t\n15:08:02.2\tlog_raw\tgps_raw\t\tsystem status\tnormal 2 28.200000 0 0\trobot status\t43.603521\t56.579476\t8.926700\t-0.766315\t-1.182755\t50.454479\t0.491000\t0.011000\n\t\n15:08:02.7\tlog_raw\tgps_raw\t#INSPVAXA,USB3,0,49.0,FINESTEERING,2107,281300.750,02000000,471d,15824;INS_ALIGNMENT_COMPLETE,INS_RTKFIXED,37.37064174008,126.72132926537,8.9257,22.3000,0.3670,0.3118,0.0263,-0.579154984,-1.155742554,37.154805631,0.4158,0.2925,0.5630,0.1150,0.0956,0.0882,0.2713,0.2501,5.0783,0f000001,0*68bc3ddc\n\tsystem status\tnormal 2 28.300000 0 0\trobot status\t43.771908\t56.773342\t8.925700\t-0.579155\t-1.155743\t50.705788\t0.493000\t0.007000\n\t\n15:08:03.2\tlog_raw\tgps_raw\t#INSPVAXA,USB3,0,45.0,FINESTEERING,2107,281301.250,02000000,471d,15824;INS_ALIGNMENT_COMPLETE,INS_RTKFIXED,37.37064333082,126.72133100341,8.9247,22.3000,0.3527,0.3031,-0.0127,-0.497881358,-1.036001571,37.376921117,0.4148,0.2915,0.5607,0.1142,0.0949,0.0876,0.2713,0.2501,5.0798,0f000001,0*cc5b3be5\n\tsystem status\tnormal 2 28.300000 0 0\trobot status\t43.925861\t56.949889\t8.924700\t-0.497881\t-1.036002\t51.052662\t0.493000\t0.017000\n\t\n15:08:03.7\tlog_raw\tgps_raw\t#INSPVAXA,USB3,0,45.0,FINESTEERING,2107,281301.750,02000000,471d,15824;INS_ALIGNMENT_COMPLETE,INS_RTKFIXED,37.37064493780,126.72133275728,8.9253,22.3000,0.3854,0.3385,0.0182,-0.710763473,-1.064044201,37.431956874,0.4148,0.2915,0.5607,0.1142,0.0949,0.0876,0.2713,0.2501,5.0798,0f000001,0*85706bc5\n\tsystem status\tnormal 2 28.200000 0 0\trobot status\t44.081216\t57.128238\t8.925300\t-0.710763\t-1.064044\t50.344284\t0.497000\t0.036000\n\t\n15:08:04.2\tlog_raw\tgps_raw\t#INSPVAXA,USB3,0,43.5,FINESTEERING,2107,281302.250,02000000,471d,15824;INS_ALIGNMENT_COMPLETE,INS_RTKFIXED,37.37064655535,126.72133453652,8.9249,22.3000,0.3513,0.3141,0.0174,-0.690110515,-1.069032412,37.638808056,0.4139,0.2898,0.5573,0.1136,0.0942,0.0868,0.2712,0.2501,5.0809,0f000001,0*cbae559e\n\tsystem status\tnormal 2 28.200000 0 0\trobot status\t44.238818\t57.307761\t8.924900\t-0.690111\t-1.069032\t50.568409\t0.495000\t0.004000\n\t\n15:08:04.7\tlog_raw\tgps_raw\t#INSPVAXA,USB3,0,43.5,FINESTEERING,2107,281302.750,02000000,471d,15824;INS_ALIGNMENT_COMPLETE,INS_RTKFIXED,37.37064813520,126.72133627740,8.9245,22.3000,0.3692,0.3319,0.0061,-0.364312615,-0.951644319,37.470597230,0.4139,0.2898,0.5573,0.1136,0.0942,0.0868,0.2712,0.2501,5.0809,0f000001,0*08b0ee33\n\tsystem status\tnormal 2 28.200000 0 0\trobot status\t44.393022\t57.483099\t8.924500\t-0.364313\t-0.951644\t50.236343\t0.496000\t0.028000\n\t\n15:08:05.2\tlog_raw\tgps_raw\t\tsystem status\tnormal 2 28.100000 0 0\trobot status\t44.527755\t57.641727\t8.922600\t-0.696399\t-0.944373\t50.297966\t0.453000\t0.086000\n\t\n15:08:05.7\tlog_raw\tgps_raw\t#INSPVAXA,USB3,0,47.5,FINESTEERING,2107,281303.750,02000000,471d,15824;INS_ALIGNMENT_COMPLETE,INS_RTKFIXED,37.37065132406,126.72133969488,8.9195,22.3000,0.3562,0.2992,-0.0320,-0.568216289,-0.963941072,36.278443582,0.4132,0.2892,0.5557,0.1134,0.0941,0.0862,0.2712,0.2500,5.0819,0f000001,0*4328ab23\n\tsystem status\tnormal 2 28.100000 0 0\trobot status\t44.695737\t57.837012\t8.919500\t-0.568216\t-0.963941\t51.084133\t0.505000\t0.026000\n\t\n15:08:06.2\tlog_raw\tgps_raw\t#INSPVAXA,USB3,0,48.0,FINESTEERING,2107,281304.250,02000000,471d,15824;INS_ALIGNMENT_COMPLETE,INS_RTKFIXED,37.37065295180,126.72134135022,8.9157,22.3000,0.3763,0.3181,0.0214,-0.552058528,-1.148423815,35.386724637,0.4128,0.2880,0.5530,0.1133,0.0938,0.0856,0.2712,0.2500,5.0827,0f000001,0*325fffc2\n\tsystem status\tnormal 2 28.100000 0 0\trobot status\t44.842364\t58.017665\t8.915700\t-0.552059\t-1.148424\t51.569904\t0.593000\t-0.120000\n\t\n15:08:06.7\tlog_raw\tgps_raw\t\tsystem status\tnormal 2 28.000000 0 0\trobot status\t44.971954\t58.184199\t8.911600\t-0.435792\t-1.120857\t53.018772\t0.379000\t0.181000\n\t\n15:08:07.2\tlog_raw\tgps_raw\t#INSPVAXA,USB3,0,49.0,FINESTEERING,2107,281305.250,02000000,471d,15824;INS_ALIGNMENT_COMPLETE,INS_RTKFIXED,37.37065630183,126.72134454819,8.9059,22.3000,0.3906,0.3004,-0.0040,-0.611614094,-1.196662940,33.418986563,0.4115,0.2871,0.5504,0.1130,0.0936,0.0850,0.2711,0.2499,5.0838,0f000001,0*b360f959\n\tsystem status\tnormal 2 28.000000 0 0\trobot status\t45.125635\t58.389465\t8.905900\t-0.611614\t-1.196663\t53.270657\t0.712000\t-0.301000\n\t\n15:08:07.7\tlog_raw\tgps_raw\t#INSPVAXA,USB3,0,49.0,FINESTEERING,2107,281305.750,02000000,471d,15824;INS_ALIGNMENT_COMPLETE,INS_RTKFIXED,37.37065799694,126.72134610571,8.8988,22.3000,0.3773,0.2695,-0.0206,-0.928046219,-1.204880173,32.568917914,0.4115,0.2871,0.5504,0.1130,0.0936,0.0850,0.2711,0.2499,5.0838,0f000001,0*cfbde854\n\tsystem status\tnormal 2 28.000000 0 0\trobot status\t45.263598\t58.577596\t8.898800\t-0.928046\t-1.204880\t54.678371\t0.436000\t0.120000\n\t\n15:08:08.2\tlog_raw\tgps_raw\t\tsystem status\tnormal 2 28.100000 0 0\trobot status\t45.383738\t58.746518\t8.892200\t-0.798731\t-1.292767\t55.600021\t0.568000\t-0.054000\n\t\n15:08:08.7\tlog_raw\tgps_raw\t#INSPVAXA,USB3,0,43.0,FINESTEERING,2107,281306.750,02000000,471d,15824;INS_ALIGNMENT_COMPLETE,INS_RTKFIXED,37.37066149033,126.72134911698,8.8812,22.3000,0.3665,0.2586,0.0068,-0.726996907,-1.292564027,31.229501347,0.4104,0.2857,0.5476,0.1128,0.0935,0.0845,0.2710,0.2498,5.0853,0f000001,0*271f73c6\n\tsystem status\tnormal 2 28.100000 0 0\trobot status\t45.530331\t58.965307\t8.881200\t-0.726997\t-1.292564\t56.382351\t0.465000\t0.054000\n\t\n15:08:09.2\tlog_raw\tgps_raw\t#INSPVAXA,USB3,0,47.5,FINESTEERING,2107,281307.250,02000000,471d,15824;INS_ALIGNMENT_COMPLETE,INS_RTKFIXED,37.37066326651,126.72135056496,8.8706,22.3000,0.3793,0.2759,-0.0087,-0.800097875,-1.188494571,30.825604162,0.4094,0.2846,0.5448,0.1127,0.0934,0.0841,0.2709,0.2497,5.0869,0f000001,0*7a768f4f\n\tsystem status\tnormal 2 28.100000 0 0\trobot status\t45.658591\t59.162435\t8.870600\t-0.800098\t-1.188495\t56.715714\t0.611000\t-0.148000\n\t\n15:08:09.7\tlog_raw\tgps_raw\t#INSPVAXA,USB3,0,47.5,FINESTEERING,2107,281307.750,02000000,471d,15824;INS_ALIGNMENT_COMPLETE,INS_RTKFIXED,37.37066506990,126.72135204695,8.8605,22.3000,0.3836,0.2569,-0.0181,-0.611818714,-1.092696034,30.573284565,0.4094,0.2846,0.5448,0.1127,0.0934,0.0841,0.2709,0.2497,5.0869,0f000001,0*79d635a4\n\tsystem status\tnormal 2 28.100000 0 0\trobot status\t45.789863\t59.362582\t8.860500\t-0.611819\t-1.092696\t56.340206\t0.414000\t0.115000\n\t\n15:08:10.2\tlog_raw\tgps_raw\t#INSPVAXA,USB3,0,46.0,FINESTEERING,2107,281308.250,02000000,471d,15824;INS_ALIGNMENT_COMPLETE,INS_RTKFIXED,37.37066685186,126.72135349986,8.8501,22.3000,0.3922,0.2593,-0.0136,-0.551675825,-0.866778153,30.503806411,0.4391,0.2876,0.5552,0.1178,0.0942,0.0847,0.2709,0.2501,5.0885,0f000001,0*c2dc3b9a\n\tsystem status\tnormal 2 28.200000 0 0\trobot status\t45.918560\t59.560352\t8.850100\t-0.551676\t-0.866778\t57.573292\t0.547000\t-0.102000\n\t\n15:08:10.7\tlog_raw\tgps_raw\t#INSPVAXA,USB3,0,46.0,FINESTEERING,2107,281308.750,02000000,471d,15824;INS_ALIGNMENT_COMPLETE,INS_RTKFIXED,37.37066865801,126.72135498437,8.8428,22.3000,0.3889,0.2874,-0.0164,-0.422088252,-1.035305211,30.456393421,0.4391,0.2876,0.5552,0.1178,0.0942,0.0847,0.2709,0.2501,5.0885,0f000001,0*b848ab12\n\tsystem status\tnormal 2 28.200000 0 0\trobot status\t46.050055\t59.760806\t8.842800\t-0.422088\t-1.035305\t56.548996\t0.542000\t-0.085000\n\t\n15:08:11.2\tlog_raw\tgps_raw\t\tsystem status\tnormal 2 28.300000 0 0\trobot status\t46.179072\t59.960946\t8.836500\t-0.409998\t-0.990799\t57.881889\t0.480000\t0.000000\n\t\n15:08:11.7\tlog_raw\tgps_raw\t#INSPVAXA,USB3,0,48.0,FINESTEERING,2107,281309.750,02000000,471d,15824;INS_ALIGNMENT_COMPLETE,INS_RTKFIXED,37.37067230614,126.72135792146,8.8292,22.3000,0.4110,0.2664,-0.0105,-0.611662697,-1.081629993,30.781825564,0.4668,0.2909,0.5674,0.1216,0.0948,0.0853,0.2709,0.2504,5.0902,0f000001,0*6b834f48\n\tsystem status\tnormal 2 28.200000 0 0\trobot status\t46.310218\t60.165691\t8.829200\t-0.611663\t-1.081630\t56.914261\t0.504000\t-0.020000\n\t\n15:08:12.2\tlog_raw\tgps_raw\t#INSPVAXA,USB3,0,46.5,FINESTEERING,2107,281310.250,02000000,471d,15824;INS_ALIGNMENT_COMPLETE,INS_RTKFIXED,37.37067411015,126.72135939117,8.8212,22.3000,0.3810,0.2710,-0.0053,-0.603115000,-1.192069099,31.016227995,0.4406,0.2869,0.5568,0.1163,0.0939,0.0842,0.2707,0.2496,5.0919,0f000001,0*94346154\n\tsystem status\tnormal 2 28.300000 0 0\trobot status\t46.440402\t60.365907\t8.821200\t-0.603115\t-1.192069\t56.870022\t0.492000\t-0.028000\n\t\n15:08:12.7\tlog_raw\tgps_raw\t#INSPVAXA,USB3,0,46.5,FINESTEERING,2107,281310.750,02000000,471d,15824;INS_ALIGNMENT_COMPLETE,INS_RTKFIXED,37.37067588400,126.72136084983,8.8127,22.3000,0.4076,0.2839,-0.0115,-0.606845317,-1.152685391,31.227730506,0.4406,0.2869,0.5568,0.1163,0.0939,0.0842,0.2707,0.2496,5.0919,0f000001,0*103e46f3\n\tsystem status\tnormal 2 28.200000 0 0\trobot status\t46.569608\t60.562777\t8.812700\t-0.606845\t-1.152685\t56.525253\t0.492000\t-0.026000\n\t\n15:08:13.2\tlog_raw\tgps_raw\t#INSPVAXA,USB3,0,46.5,FINESTEERING,2107,281311.250,02000000,471d,15824;INS_ALIGNMENT_COMPLETE,INS_RTKFIXED,37.37067773364,126.72136238370,8.8047,22.3000,0.4077,0.2865,0.0068,-0.584908191,-1.091980758,31.544161154,0.4259,0.2849,0.5501,0.1143,0.0937,0.0835,0.2705,0.2492,5.0936,0f000001,0*c1eb006b\n\tsystem status\tnormal 2 28.200000 0 0\trobot status\t46.705476\t60.768057\t8.804700\t-0.584908\t-1.091981\t56.063690\t0.492000\t-0.020000\n\t\n15:08:13.7\tlog_raw\tgps_raw\t#INSPVAXA,USB3,0,46.5,FINESTEERING,2107,281311.750,02000000,471d,15824;INS_ALIGNMENT_COMPLETE,INS_RTKFIXED,37.37067959251,126.72136394573,8.7964,22.3000,0.4141,0.2904,-0.0295,-0.451303180,-1.068459528,31.726821051,0.4259,0.2849,0.5501,0.1143,0.0937,0.0835,0.2705,0.2492,5.0936,0f000001,0*f5652221\n\tsystem status\tnormal 2 28.200000 0 0\trobot status\t46.843838\t60.974363\t8.796400\t-0.451303\t-1.068460\t55.266247\t0.494000\t-0.023000\n\t\n15:08:14.2\tlog_raw\tgps_raw\t#INSPVAXA,USB3,0,48.5,FINESTEERING,2107,281312.250,02000000,471d,15824;INS_ALIGNMENT_COMPLETE,INS_RTKFIXED,37.37068138188,126.72136546046,8.7891,22.3000,0.3907,0.2897,-0.0164,-0.536773748,-1.064691543,31.954893776,0.4173,0.2841,0.5455,0.1136,0.0938,0.0834,0.2704,0.2490,5.0951,0f000001,0*3086f5e7\n\tsystem status\tnormal 2 28.200000 0 0\trobot status\t46.978010\t61.172954\t8.789100\t-0.536774\t-1.064692\t55.577579\t0.495000\t-0.019000\n\t\n15:08:14.7\tlog_raw\tgps_raw\t#INSPVAXA,USB3,0,48.5,FINESTEERING,2107,281312.750,
